vi "例程05-字符串.vi"() -> ()   [LabVIEW 2018]
panel:
  out "数字":i32
  in  "数字字符串":string
  out "连接的字符串 2":string
  out "连接的字符串":string
  out "字符串长度":dbl
  in  "字符串":string
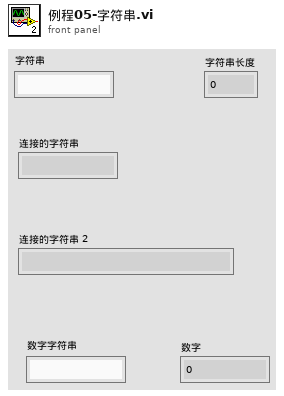
[diagram p1: front panel]
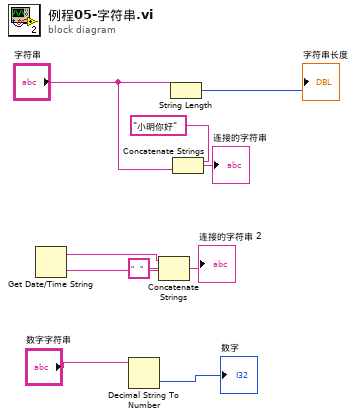
[diagram p0: block diagram]
diagram:
  n1 = Get Date/Time String() -> (date string=w6:string, time string=w3:string)  [unwired: 3 in]
  n2 = Decimal String To Number(string="数字字符串") -> (number=→"数字":i32)  [unwired: 2 in, 1 out]
  n3 = Concatenate Strings(w6, "   " ("字符串"), w3) -> (→"连接的字符串 2":string)
  n4 = String Length(string="字符串") -> (length=→"字符串长度":i32)
  n5 = Concatenate Strings("小明你好" ("字符串"), "字符串") -> (→"连接的字符串":string)
